vi "TCP 클라.vi"() -> ()   [LabVIEW 2018]
panel:
  in  "정지":bool
  out "웨이브폼 그래프":dbl[](graph)
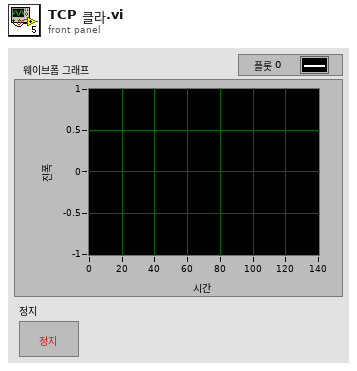
[diagram p1: front panel]
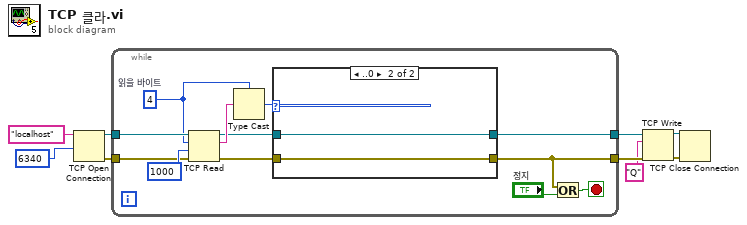
[diagram p0: block diagram]
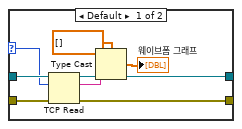
[diagram p2: hidden frame]
diagram:
  n1 = TCP Open Connection(address="localhost" ("주소"), remote port or service name=u16 6340 ("포트")) -> (connection ID=w6:refnum<k5>, error out=w7:errorcluster)  [unwired: 3 in]
  n2 = while {
    tunnel: w7 -> [w20]
    tunnel: w6 -> [w19]
    tunnel: [w12] -> w4
    tunnel: [w13] -> w5
    stop <- w11 stop-if-true
    w17 = 4  # 읽을 바이트
    n3 = TCP Read(connection ID=w19, bytes to read=w17, error in (no error)=w20, 9:1000 ("타임아웃 ms (25000)")) -> (connection ID out=w14:refnum<k5>, data out=w18:string, error out=w15:errorcluster)  [unwired: 1 in]
    n4 = Type Cast(type=w17, x=w18) -> (*(type *) &x=w16:i32)
    n5 = case shown="..0" w16 {
      selector: w16 -> [w22 _]
      tunnel: w15 -> [w27 w31]
      tunnel: [w26 w31] -> w12
      tunnel: w14 -> [w29 w30]
      tunnel: [w28 w30] -> w13
      frame Default {
        n6 = TCP Read(connection ID=w29, bytes to read=w22, error in (no error)=w27) -> (connection ID out=w28:refnum<k5>, data out=w24:string, error out=w26:errorcluster)  [unwired: 2 in]
        n7 = Type Cast(type=dbl[] [], x=w24) -> (*(type *) &x=→"웨이브폼 그래프":dbl[])
      }
      frame ..0 {
      }
    }
    n8 = Or(x=w12, y="정지") -> (x .or. y?=w11:bool)
  }
  n9 = TCP Write(connection ID=w5, data in="Q" ("데이터 입력"), error in (no error)=w4) -> (connection ID out=w2:refnum<k5>, error out=w3:errorcluster)  [unwired: 1 in, 1 out]
  n10 = TCP Close Connection(connection ID=w2, error in (no error)=w3) -> ()  [unwired: 1 in, 2 out]
